vi "Write_ini_file.vi"() -> ()   [LabVIEW 2018]
uses:
  <vilib>/Utility/config.llb/Write Key (I32).vi
  <vilib>/Utility/config.llb/Write Key (U32).vi
  <vilib>/Utility/config.llb/NI_LVConfig.lvlib
panel:
  in  "Active Layer":i32(ring) items=["Layer 0", "Layer 1", "Layer 2", "Layer 3"]
  in  "Pulley Position":u32(slide)=40 max=51 step=1 scale=0.0..51.0
  out "error out (config.ini file)":errorcluster
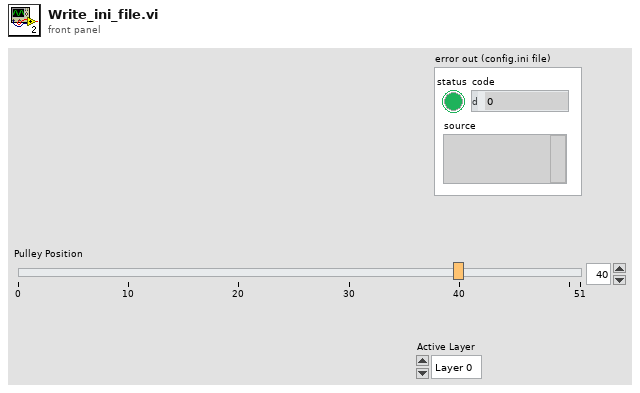
[diagram p1: front panel]
types:
  T1 = typedef "NI_LVConfig.lvlib/Config Data RefNum.ctl" = refnum<k1>
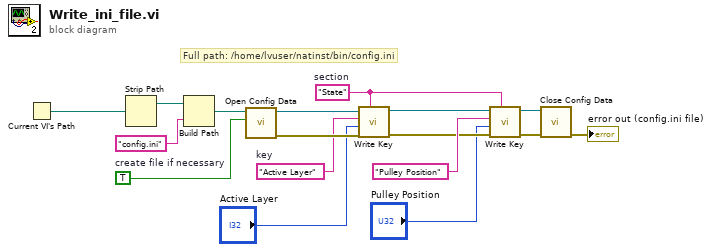
[diagram p0: block diagram]
diagram:
  w10 = "Active Layer"  # key
  w8 = "State"  # section
  w13 = TRUE  # create file if necessary
  # "Full path: /home/lvuser/natinst/bin/config.ini"
  n1 = Current VI's Path() -> (path=w16:path)
  n2 = Strip Path(path=w16) -> (stripped path=w17:path)  [unwired: 1 out]
  n3 = Build Path(base path=w17, name or relative path="config.ini") -> (appended path=w14:path)
  n4 = call <vilib>:"Open Config Data.vi"("create file if necessary (T)"=w13, "configuration file path"=w14) -> ("error out"=w11:errorcluster, "refnum"=w12:T1)  [unwired: 7 in, 1 out]
  n5 = call-poly <vilib>:"Write Key.vi"("section"=w8, "error in (no error)"=w11, "value"="Active Layer", "key"=w10, "refnum"=w12) -> ("error out"=w6:errorcluster, "refnum out"=w9:T1)  [unwired: 4 in, 1 out]
  n6 = call-poly <vilib>:"Write Key.vi"("section"=w8, "error in (no error)"=w6, "value"="Pulley Position", "key"="Pulley Position", "refnum"=w9) -> ("error out"=w5:errorcluster, "refnum out"=w4:T1)  [unwired: 4 in, 1 out]
  n7 = call <vilib>:"Close Config Data.vi"("error in (no error)"=w5, "refnum"=w4) -> ("error out"=→"error out (config.ini file)":errorcluster)  [unwired: 8 in, 1 out]
